vi "Any_Ref_enthalpy_funct_TP_REFPROP10.vi"(1 "Input Temperature [C]":dbl, 2 "Input Pressure [kPa]":dbl, 3 "error in (no error)":errorcluster, 4 "?":path=path "C:/Users/ASITest/Desktop/REFPROP", 6 "Fluidofinterest":string="R134a.FLD") -> (7 "Enthalpy [kJ/kg]":dbl, 8 "Entropy":dbl, 9 "Density":dbl, 10 "error out":errorcluster)   [LabVIEW 2016]
doc: "Return refrigerant enthalpy [kJ/kg] for specified refrigerant, input pressure [kPa] and temperature [C]"
panel:
  out "name out":string
  out "data":string[][](table)=[["0", "T", "40.917420"], ["1", "P", "632.917420"], ["2", "H", "466.332574"], ["3", "S", "2.054657"], ["4", "DV", "18.926081"], ["5", "DL", "18.926081"], ["6", "E", "432.891028"], ["7", "CV", "0.758226"], ["8", "CP", "0.924261"], ["9", "W", "194.299169"], ["10", "Q", "998.000000"]]
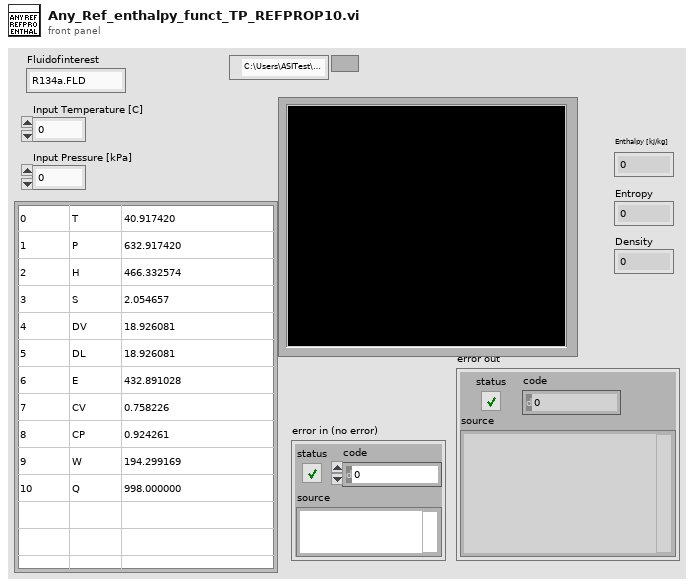
[diagram p1: front panel]
types:
  T1 = enum16{"0", "PS", "HS", "T", "P", "TP", "TH", "TS", "PH", "PQ", "TQ"}
  T2 = typedef "Mixture Composition cluster_d.ctl" = cluster{"Mixture Name":string, "Molecular weight (g/mol)":dbl, "Critical temperature (K)":dbl, "Critical Pressure (kPa)":dbl, "Critical Density (mol/L)":dbl, "# Components":i32, "Fluid File Paths":path[], "Component molar fractions":dbl[], "Refprop Main Directory":path, "DLL Version Number":dbl}
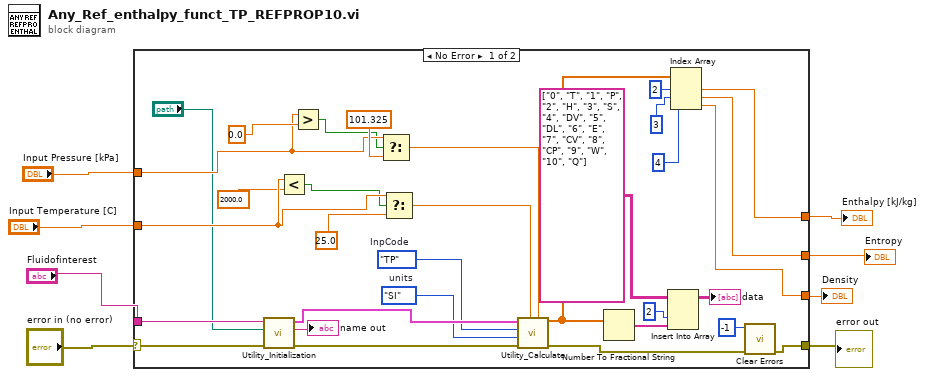
[diagram p0: block diagram]
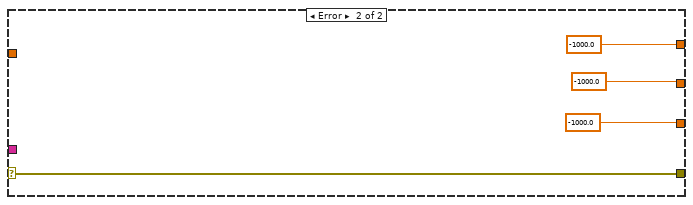
[diagram p2: hidden frame]
diagram:
  n1 = case shown="No Error" "error in (no error)" {
    selector: "error in (no error)" -> [w33 w44]
    tunnel: [w25 w44] -> w7
    tunnel: [w28 -1000.0 ("Numeric")] -> w6
    tunnel: "Input Pressure [kPa]" -> [w11 _]
    tunnel: "Fluidofinterest" -> [w27 _]
    tunnel: "Input Temperature [C]" -> [w15 _]
    tunnel: [w21 -1000.0 ("Numeric")] -> w1
    tunnel: [w20 -1000.0 ("Numeric")] -> w2
    frame No Error {
      w31 = T1."TP"  # InpCode
      w32 = enum16{"SI", "IP"}."SI"  # units
      n2 = call "Utility_Initialization.vi"("error in (no error)"=w33, "path"="?", "Fluidofinterest"=w27) -> ("error out"=w36:errorcluster, "name out"=→"name out":string, "Mixure Cluster out"=w34:T2)  [unwired: 6 in]
      n3 = Less?(x=w15, y=2000.0) -> (x < y?=w14:bool)
      n4 = Greater?(x=w11, y=0.0) -> (0:w10:bool)
      n5 = Select(t=w11, s=w10, f=101.325) -> (s? t:f=w18:dbl)
      n6 = Select(t=w15, s=w14, f=25.0) -> (s? t:f=w16:dbl)
      n7 = call "Utility_Calculate.vi"("input_2"=w18, "input_1"=w16, "error in"=w36, "units"=w32, "InpCode"=w31, "Mixure Cluster"=w34) -> ("error out"=w26:errorcluster, "dataout"=w30:dbl[])  [unwired: 3 in]
      n8 = Number To Fractional String(number=w30) -> (F-format string=w39:string[])  [unwired: 3 in]
      n9 = Insert Into Array(array=string[][] [["0", "T"], ["1", "P"], ["2", "H"], ["3", "S"], ["4", "DV"], ["5", "DL"], ["6", "E"], ["7", "CV"], ["8", "CP"], ["9", "W"], ["10", "Q"]] ("数组"), index (col)=2 ("禁用的索引 (列)"), new element=w39) -> (→"data":string[][])  [unwired: 1 in]
      n10 = Index Array(array=w30, index #1=2 ("index"), index #2=3 ("index"), index #3=4 ("index")) -> (element #1=w28:dbl, element #2=w21:dbl, element #3=w20:dbl)
      n11 = call <vilib>:"Clear Errors.vi"("error in (no error)"=w26, "specific error code to clear (0: all)"=-1) -> ("error out"=w25:errorcluster)  [unwired: 4 in, 1 out]
    }
    frame Error {
    }
  }
  "error out" <- w7
  "Enthalpy [kJ/kg]" <- w6
  "Entropy" <- w1
  "Density" <- w2
